vi "ma_SML Peak-hold Averaging (real input).vi"(0 "x":dbl[](array[numeric]) format="%.2f", 1 "reset?":bool) -> (2 "y":dbl[](array[numeric]) format="%.2f", 3 "averages sofar":dbl, 4 "data ready?":bool)   [LabVIEW 2020, in "NI_MAPro.lvlib"]
uses:
  NI_MAPro.lvlib
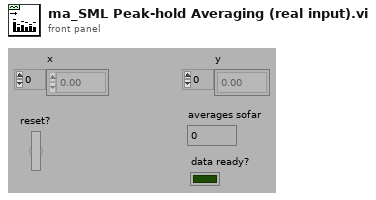
[diagram p1: front panel]
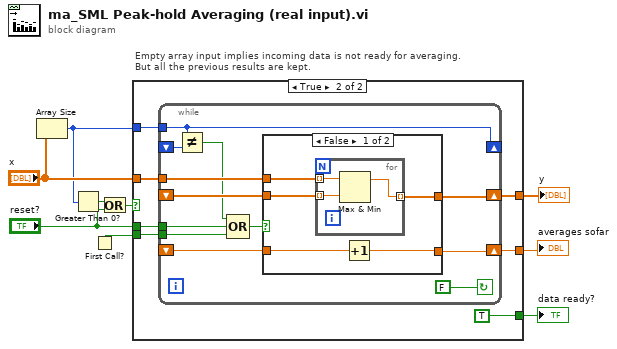
[diagram p0: block diagram]
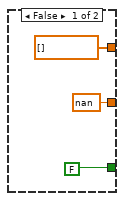
[diagram p2: hidden frame]
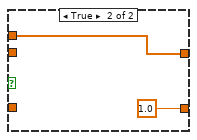
[diagram p3: hidden frame]
diagram:
  # "Empty array input implies incoming data is not ready for averaging.\nBut all the previous results are kept."
  n1 = Array Size(array="x") -> (size(s)=w5:i32)
  n2 = Greater Than 0?(x=w5) -> (x > 0?=w6:bool)
  n3 = First Call?() -> (First Call?: T/F=w1:bool)
  n4 = Or(x=w6, y="reset?") -> (x .or. y?=w4:bool)
  n5 = case shown="True" w4 {
    tunnel: "x" -> [_ w19]
    tunnel: w5 -> [_ w18]
    tunnel: "reset?" -> [_ w17]
    tunnel: [dbl[] [] ("x") w16] -> w8
    tunnel: [nan w15] -> w7
    tunnel: [FALSE TRUE] -> w3
    tunnel: w1 -> [_ w13]
    frame False {
    }
    frame True {
      n6 = while {
        tunnel: w13 -> [w20]
        shift-left: _ -> [w26]
        shift-right: [w27] -> w15
        shift-left: _ -> [w28]
        shift-right: [w29] -> w16
        tunnel: w17 -> [w22]
        tunnel: w18 -> [w21]
        tunnel: w19 -> [w30]
        shift-left: _ -> [w31]
        shift-right: [w21] -> _
        stop <- FALSE continue-if-true
        n7 = Not Equal?(x=w21, y=w31) -> (x != y?=w23:bool)
        n8 = Compound Arithmetic op=OR(w23, w22, w20) -> (w24:bool)
        n9 = case shown="False" w24 {
          tunnel: [w34 w41] -> w29
          tunnel: w30 -> [w36 w41]
          tunnel: w28 -> [w35 _]
          tunnel: [w32 1.0] -> w27
          tunnel: w26 -> [w33 _]
          frame False {
            n10 = for {
              tunnel: w36 -> [w39] mode=indexing
              tunnel: w35 -> [w38] mode=indexing
              tunnel: [w37] -> w34 mode=indexing
              n11 = Max & Min(x=w39, y=w38) -> (max(x,y)=w37:dbl)  [unwired: 1 out]
            }
            n12 = Increment(x=w33) -> (x+1=w32:dbl)
          }
          frame True {
          }
        }
      }
    }
  }
  "y" <- w8
  "averages sofar" <- w7
  "data ready?" <- w3
